vi "Weather Station UI.vi"(10 "하위 리미트":dbl=10.0, 11 "상위 리미트":dbl=30.0) -> (1 "경고":string, 2 "온도 히스토리":dbl(graph))   [LabVIEW 2010]
doc: "이는 기상 관측기 프로젝트의 주요 VI입니다. 온도 경고 시스템을 위한 사용자 인터페이스를 포함합니다.\n\n사용자 입력: 최대 온도, 최소 온도, 온도 단위.\n출력: 현재 온도, 경고 상태"
uses:
  Supporting Files/Weather Station States.ctl
panel:
  in  "날씨 데이터":dynamicdata(graph)
  in  "정지":bool
  in  "풍속 상위 리미트":dbl(slide)=50.0 scale=0.0..100.0
  out "풍속 히스토리":dbl(graph)
  # "섭씨"
  # "온도 범위"
  # "열사병"
  # "동상"
  # "kph"
  # "최대 안전 풍속"
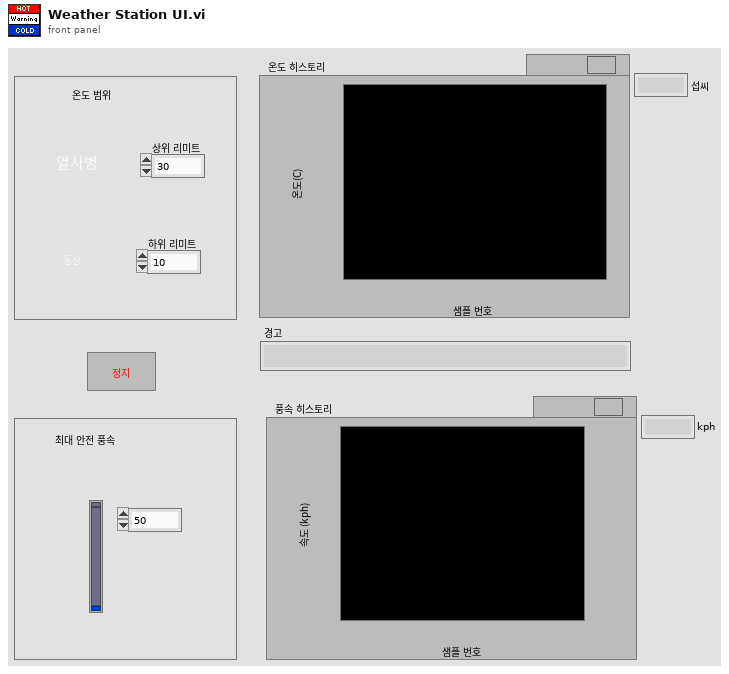
[diagram p1: front panel]
types:
  T1 = cluster{"온도":dbl, "온도 상위 리미트":dbl, "온도 하위 리미트":dbl, "풍속":dbl, "풍속 상위 리미트":dbl, "경고":string, "시간":dbl}
  T2 = typedef "Weather Station States.ctl" = enum16{"분석", "UI 처리", "경고 설정", "데이터 로그", "정지"}
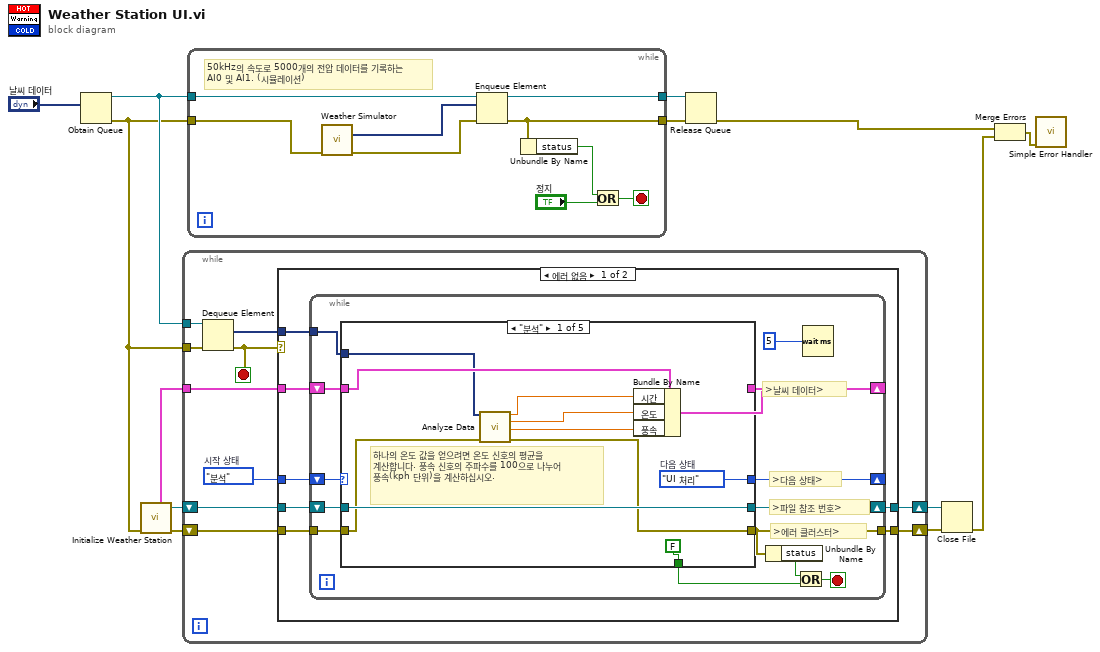
[diagram p0: block diagram]
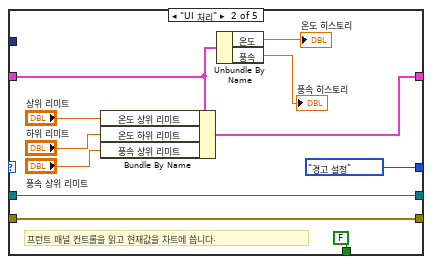
[diagram p2: hidden frame]
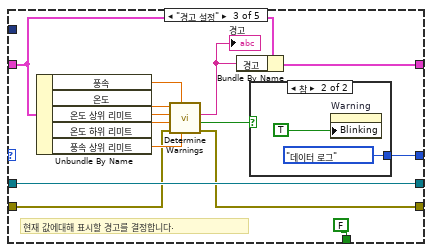
[diagram p3: hidden frame]
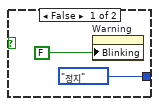
[diagram p4: hidden frame]
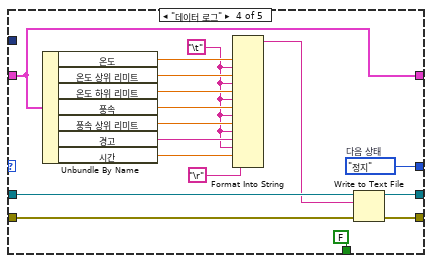
[diagram p5: hidden frame]
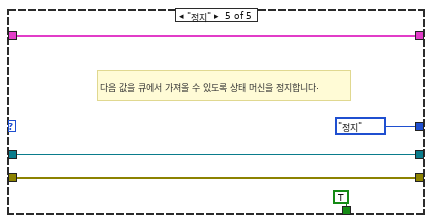
[diagram p6: hidden frame]
diagram:
  n1 = Obtain Queue ("큐 얻기")(element data type="날씨 데이터") -> (queue out=w10:refnum<queue>, error out=w1:errorcluster)  [unwired: 3 in, 2 out]
  n2 = call "Initialize Weather Station.vi"("에러 입력(에러 없음)"=w1) -> ("에러 출력"=w2:errorcluster, "파일 참조 번호"=w3:refnum<file>, "날씨 데이터"=w13:T1)  [unwired: 8 out]
  n3 = while "While 루프" {
    tunnel: w13 -> [w22]
    tunnel: w10 -> [w21]
    tunnel: w1 -> [w20]
    shift-right: [w23] -> w6
    shift-left: w3 -> [w19]
    shift-right: [w15] -> w5
    shift-left: w2 -> [w16]
    stop <- w18 stop-if-true
    w14 = Weather_Station_States."분석"  # 시작 상태
    n4 = Dequeue Element ("원소를 큐에서 제거")(queue=w21, error in (no error)=w20) -> (element=w17:dynamicdata, error out=w18:errorcluster)  [unwired: 3 out]
    n5 = case "케이스 구조" shown="에러 없음" w18 {
      tunnel: [w30 w106] -> w23
      tunnel: w22 -> [w29 _]
      tunnel: w19 -> [w28 w106]
      tunnel: w17 -> [w27 _]
      tunnel: w16 -> [w25 w107]
      tunnel: [w26 w107] -> w15
      tunnel: w14 -> [w24 _]
      frame No Error {
        n6 = while {
          shift-right: [w43] -> _
          shift-left: w24 -> [w35]
          shift-right: [w32] -> w30
          shift-left: w28 -> [w42]
          shift-right: [w36] -> _
          shift-left: w29 -> [w39]
          tunnel: w27 -> [w34]
          tunnel: [w33] -> w26
          tunnel: w25 -> [w31]
          stop <- w41 stop-if-true
          # ">에러 클러스터>"
          # ">날씨 데이터>"
          # ">파일 참조 번호>"
          # ">다음 상태>"
          n7 = case shown="\"분석\"" w35 {
            tunnel: [w54 Weather_Station_States."경고 설정" ("Next State") w78 w100 Weather_Station_States."정지" ("Next State")] -> w43
            tunnel: [w44 w56 w69 w97 w101] -> w33
            tunnel: w42 -> [w50 w55 w76 w96 w102]
            tunnel: [w51 w65 w66 w94 w103] -> w36
            tunnel: w39 -> [w52 w62 w77 w94 w103]
            tunnel: [FALSE ("stop") FALSE ("stop") FALSE ("stop") FALSE ("stop") TRUE ("stop")] -> w38
            tunnel: w34 -> [w49 _ _ _ _]
            tunnel: [w50 w55 w76 w98 w102] -> w32
            tunnel: w31 -> [w48 w56 w70 w84 w101]
            frame "분석" {
              w54 = Weather_Station_States."UI 처리"  # 다음 상태
              # "하나의 온도 값을 얻으려면 온도 신호의 평균을 계산합니다. 풍속 신호의 주파수를 100으로 나누어 풍속(kph 단위)을 계산하십시오."
              n8 = call "Analyze Data.vi"("날씨 데이터"=w49, "에러 입력"=w48) -> ("시간"=w47:dbl, "온도"=w46:dbl, "풍속"=w45:dbl, "에러 출력"=w44:errorcluster)  [unwired: 2 in, 8 out]
              n9 = Bundle By Name(cluster=w52, "시간"=w47, "온도"=w46, "풍속"=w45) -> (w51:T1)
            }
            frame "UI 처리" {
              # "프런트 패널 컨트롤을 읽고 현재값을 차트에 씁니다."
              n10 = Bundle By Name(cluster=w62, "온도 상위 리미트"="상위 리미트", "온도 하위 리미트"="하위 리미트", "풍속 상위 리미트"="풍속 상위 리미트") -> (w65:T1)
              n11 = Unbundle By Name(w62) -> ("온도"=→"온도 히스토리":dbl, "풍속"=→"풍속 히스토리":dbl)
            }
            frame "경고 설정" {
              # "현재 값에대해 표시할 경고를 결정합니다."
              n12 = Unbundle By Name(w77) -> ("풍속"=w75:dbl, "온도"=w74:dbl, "온도 상위 리미트"=w73:dbl, "온도 하위 리미트"=w72:dbl, "풍속 상위 리미트"=w71:dbl)
              n13 = call "Determine Warnings.vi"("최대 풍속"=w71, "현재 풍속"=w75, "에러 입력(에러 없음)"=w70, "최저 온도"=w72, "최고 온도"=w73, "현재 온도"=w74) -> ("에러 출력"=w69:errorcluster, "경고?"=w68:bool, "경고 텍스트"=w67:string)  [unwired: 3 out]
              "경고" <- w67
              n14 = Bundle By Name(cluster=w77, "경고"=w67) -> (w66:T1)
              n15 = case shown="참" w68 {
                tunnel: [Weather_Station_States."정지" ("Next State") Weather_Station_States."데이터 로그" ("Next State")] -> w78
                frame False {
                  n16 = property on="Warning" class="Str"("Blinking"=FALSE) -> ()  [unwired: 2 in, 2 out]
                }
                frame True {
                  n17 = property on="Warning" class="Str"("Blinking"=TRUE) -> ()  [unwired: 2 in, 2 out]
                }
              }
            }
            frame "데이터 로그" {
              w86 = "\t"
              w100 = Weather_Station_States."정지"  # 다음 상태
              n18 = Unbundle By Name(w94) -> ("온도"=w93:dbl, "온도 상위 리미트"=w92:dbl, "온도 하위 리미트"=w91:dbl, "풍속"=w90:dbl, "풍속 상위 리미트"=w89:dbl, "경고"=w88:string, "시간"=w87:dbl)
              n19 = Format Into String(w93, w86, w92, w86, w91, w86, w90, w86, w89, w86, w88, w86, w87, "\r") -> (resulting string=w95:string)  [unwired: 3 in, 1 out]
              n20 = Write to Text File(file (use dialog)=w96, text=w95, error in=w84) -> (refnum out=w98:refnum<file>, error out=w97:errorcluster)  [unwired: 2 out]
            }
            frame "정지" {
              # "다음 값을 큐에서 가져올 수 있도록 상태 머신을 정지합니다."
            }
          }
          n21 = Unbundle By Name(w33) -> ("status"=w40:bool)
          n22 = Or(x=w40, y=w38) -> (x .or. y?=w41:bool)
          n23 = Wait (ms)(milliseconds to wait=u32 5 ("y")) -> ()  [unwired: 1 out]
        }
      }
      frame Error {
      }
    }
  }
  n24 = while "While 루프" {
    tunnel: w10 -> [w116]
    tunnel: w1 -> [w110]
    tunnel: [w113] -> w12
    tunnel: [w115] -> w11
    stop <- w111 stop-if-true
    # "50kHz의 속도로 5000개의 전압 데이터를 기록하는 AI0 및 AI1. (시뮬레이션)"
    n25 = call "Weather Simulator.vi"("에러 입력(에러 없음)"=w110) -> ("웨이브폼 그래프"=w108:dynamicdata, "에러 출력"=w109:errorcluster)  [unwired: 13 out]
    n26 = Enqueue Element ("원소를 큐에 추가")(queue=w116, element=w108, error in (no error)=w109) -> (queue out=w115:refnum<queue>, error out=w113:errorcluster)  [unwired: 2 out]
    n27 = Unbundle By Name ("이름으로 풀기")(w113) -> ("status"=w112:bool)
    n28 = Or(x=w112, y="정지") -> (x .or. y?=w111:bool)
  }
  n29 = Release Queue ("큐 해제")(queue=w11, error in (no error)=w12) -> (error out=w8:errorcluster)  [unwired: 3 out]
  n30 = Close File ("파일 닫기")(refnum=w6, error in=w5) -> (error out=w4:errorcluster)  [unwired: 1 out]
  n31 = Merge Errors(w8, w4) -> (w7:errorcluster)
  n32 = call <vilib>:"Simple Error Handler.vi"("error in (no error)"=w7) -> ()  [unwired: 1 in, 8 out]
